vi "Communication Tests - ClientToServer.vi"(8 "error in (no error)":errorcluster) -> (0 "error out":errorcluster)   [LabVIEW 2017]
uses:
  Support/Communication Clients/Communication Clients/Communication Clients Messages/Send Message Msg/Send Message Msg.lvclass/Send Message Msg.ctl
  <vilib>/ActorFramework/Message Enqueuer/Message Enqueuer.lvclass/Message Enqueuer.ctl
  src/LabVIEW/vi.lib/BenjaminR/Build Farm/Actors/Communication/Connection Listener/Connection Listener/Connection Listener.lvclass/Connection Listener.ctl
  src/LabVIEW/vi.lib/BenjaminR/Build Farm/Actors/Communication/Connection Listener/Connection Listener/Read Msg Update.vi
  <vilib>/ActorFramework/Message Enqueuer/Enqueue.vi
  Support/Communication Clients/Communication Clients/Communication Clients Messages/Send Message Msg/Send Message Msg.lvclass
  C:/Program Files (x86)/National Instruments/LabVIEW 2017/vi.lib/ActorFramework/Message/Message.lvclass
  src/LabVIEW/vi.lib/BenjaminR/Build Farm/Actors/Communication/Connection Listener/Connection Listener/Connection Listener.lvclass
  C:/Program Files (x86)/National Instruments/LabVIEW 2017/vi.lib/ActorFramework/Actor/Actor.lvclass
  <vilib>/ActorFramework/Stop Msg/Stop Msg.lvclass
  <vilib>/ActorFramework/Message Priority Queue/Priority Enqueue.vi
  <vilib>/addons/_JKI Toolkits/Caraya/classes/Assert/Assert True.vi
  Support/Communication Clients/Communication Clients/Communication Clients/Communication Clients.lvclass
  <vilib>/ActorFramework/Actor/Actor.lvclass
  <vilib>/addons/_JKI Toolkits/Caraya/classes/Test/Test.lvclass
  <vilib>/addons/_JKI Toolkits/Caraya/classes/Assert/Assert.lvclass
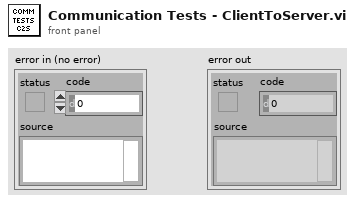
[diagram p1: front panel]
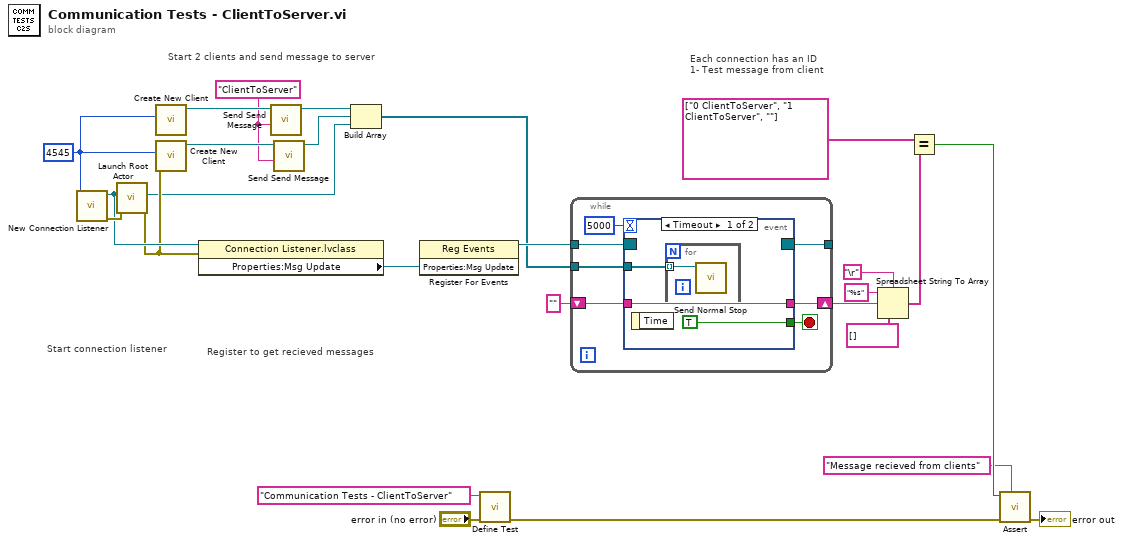
[diagram p0: block diagram]
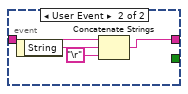
[diagram p2: hidden frame]
diagram:
  w15 = "ClientToServer" ("Message")
  w25 = u16 4545 ("Port")
  # "Start 2 clients and send message to server"
  # "Register to get recieved messages"
  # "Start connection listener"
  # "Each connection has an ID\n1- Test message from client"
  n1 = call "New Connection Listener.vi"("Port"=w25) -> ("error out"=w26:errorcluster, "Connection Listener out"=w24:refnum<class "Connection Listener.lvclass">)  [unwired: 9 in]
  n2 = call <vilib>:"Launch Root Actor.vi"("error in (no error)"=w26, "Actor"=w24) -> ("error out"=w20:errorcluster, "Actor's Enqueuer"=w8:refnum<class "Message Enqueuer.lvclass">)  [unwired: 8 in]
  n3 = call "Create New Client.vi"("Port"=w25) -> ("Message Enqueuer out"=w19:refnum<class "Message Enqueuer.lvclass">)  [unwired: 9 in, 1 out]
  n4 = call "Create New Client.vi"("error in (no error)"=w20, "Port"=w25) -> ("Message Enqueuer out"=w17:refnum<class "Message Enqueuer.lvclass">)  [unwired: 8 in, 1 out]
  n5 = property class="Connection Listener.lvclass"(reference=w24, error in=w20) -> ("Properties:Msg Update"=w23:refnum<user-event>)  [unwired: 2 out]
  n6 = call "Send Send Message.vi"("Message"=w15, "Message Enqueuer"=w19) -> ("Message Enqueuer out"=w18:refnum<class "Message Enqueuer.lvclass">)  [unwired: 8 in, 1 out]
  n7 = call "Send Send Message.vi"("Message"=w15, "Message Enqueuer"=w17) -> ("Message Enqueuer out"=w16:refnum<class "Message Enqueuer.lvclass">)  [unwired: 8 in, 1 out]
  n8 = Build Array(w18, w16, w8) -> (w5:refnum<class "Message Enqueuer.lvclass">[])
  n9 = register-events(w23) -> (reference out=w22:refnum<event-registration>)  [unwired: 2 in, 1 out]
  n10 = call <vilib>:"Define Test.vi"("error in (no error)"="error in (no error)", "Label (VI Title)"="Communication Tests - ClientToServer") -> ("error out"=w4:errorcluster)  [unwired: 9 in]
  n11 = while {
    tunnel: w22 -> [w33]
    shift-right: [w30] -> w14
    shift-left: "" -> [w31]
    tunnel: [w28] -> _
    tunnel: w5 -> [w27]
    stop <- w32 stop-if-true
    n12 = event shown="[0] Timeout" {
      selector: w33 -> [_ _]
      dyn-events: [_ _] -> w28
      timeout: 5000 -> [_ _]
      tunnel: [TRUE ("Discard?") _] -> w32
      tunnel: w31 -> [w36 w41]
      tunnel: [w36 w40] -> w30
      tunnel: w27 -> [w34 _]
      event Timeout {
        n13 = event-data() -> ()  [unwired: 1 in, 1 out]
        n14 = for {
          tunnel: w34 -> [w37] mode=indexing
          n15 = call <vilib>:"Send Normal Stop.vi"("Message Enqueuer"=w37) -> ()  [unwired: 10 in, 1 out]
        }
      }
      event User Event {
        n16 = event-data() -> ("String"=w39:string)  [unwired: 1 in]
        n17 = Concatenate Strings(w41, w39, "\r") -> (w40:string)
      }
    }
  }
  n18 = Spreadsheet String To Array(delimiter (Tab)="\r", format string="%s", spreadsheet string=w14, array type (2D Dbl)=string[] []) -> (array=w10:string[])
  n19 = Equal?(x=string[] ["0 ClientToServer", "1 ClientToServer", ""] ("array"), y=w10) -> (x = y?=w3:bool)
  n20 = call-poly <vilib>:"Assert.vi"("Label"="Message recieved from clients", "error in (no error)"=w4, "True?"=w3) -> ("error out"=→"error out":errorcluster)  [unwired: 8 in]
